vi "Check if Valid and Generate Error.vi"(5 "generate error if invalid (F)":bool, 7 "chain levels to remove (2)":i32=2, 8 "error in (no error)":errorcluster, 11 "sentence":string) -> (0 "error out":errorcluster, 3 "valid sentence":bool)   [LabVIEW 2011, in "u-blox 5 Series.lvlib"]
uses:
  u-blox 5 Series.lvlib
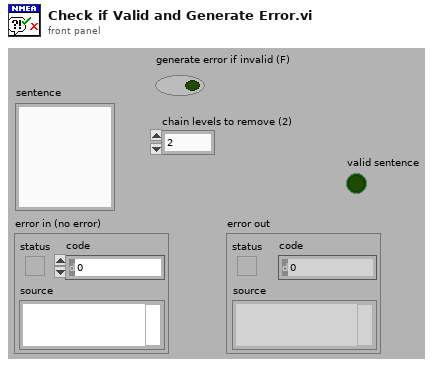
[diagram p1: front panel]
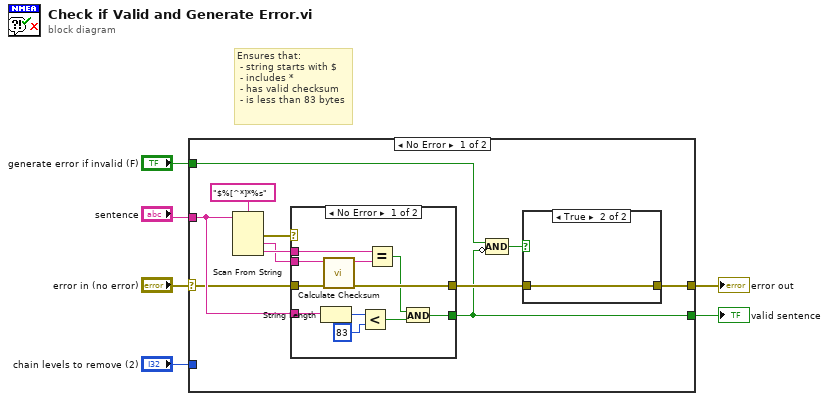
[diagram p0: block diagram]
diagram:
  # "Ensures that: \n - string starts with $ \n - includes * \n - has valid checksum\n - is less than 83 bytes"
  n1 = case shown="No Error" "error in (no error)" {
    selector: "error in (no error)" -> [w12 w32]
    tunnel: "sentence" -> [w15 _]
    tunnel: [w7 w32] -> w3
    tunnel: [w9 _] -> w4
    tunnel: "generate error if invalid (F)" -> [w10 _]
    tunnel: "chain levels to remove (2)" -> [_ _]
    frame No Error {
      n2 = Scan From String(format string="$%[^*]*%s", input string=w15) -> (error out=w13:errorcluster, output 1=w14:string, output 2=w16:string)  [unwired: 2 in, 4 out]
      n3 = case shown="No Error" w13 {
        tunnel: w16 -> [w30 _]
        tunnel: w15 -> [w29 _]
        tunnel: [w20 _] -> w9
        tunnel: w14 -> [w26 _]
        tunnel: [w24 w31] -> w11
        tunnel: w12 -> [w23 w31]
        frame No Error {
          n4 = String Length(string=w29) -> (length=w28:i32)
          n5 = call "Calculate Checksum.vi"("error in (no error)"=w23, "string"=w26) -> ("error out"=w24:errorcluster, "checksum"=w25:string)  [unwired: 6 in]
          n6 = Less?(x=w28, y=83) -> (x < y?=w22:bool)
          n7 = Equal?(x=w30, y=w25) -> (x = y?=w21:bool)
          n8 = And(x=w21, y=w22) -> (x .and. y?=w20:bool)
        }
        frame Error {
        }
      }
      n9 = Compound Arithmetic op=AND(w10, invert w9) -> (w8:bool)
      n10 = case shown="True" w8 {
        tunnel: w11 -> [w18 w19]
        tunnel: [w18 w19] -> w7
        frame False {
        }
        frame True {
        }
      }
    }
    frame Error {
    }
  }
  "valid sentence" <- w4
  "error out" <- w3
